vi "Get Autocomplete Search String.vi"(7 "String in":refnum<vi>, 11 "Autocomplete State in":T1) -> (2 "Search String":string, 3 "Autocomplete State out":T1)   [LabVIEW 2020, in "Output Sequencer.lvlib" / "Settings UI.lvclass"]
uses:
  Settings UI.lvclass
  Types/Autocomplete State.ctl
  Output Sequencer/Globals/Global Strings.vi
  Output Sequencer/Output Sequencer.lvclass
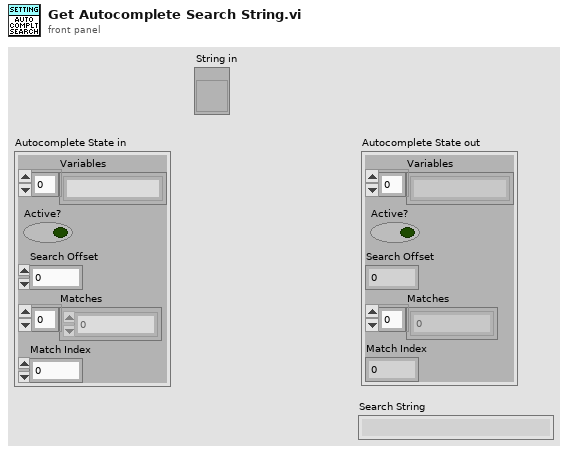
[diagram p1: front panel]
types:
  T1 = typedef "Output Sequencer.lvlib/Settings UI.lvclass/Autocomplete State.ctl" = cluster{"Variables":string[], "Active?":bool, "Search Offset":i32, "Matches":i32[], "Match Index":i32}
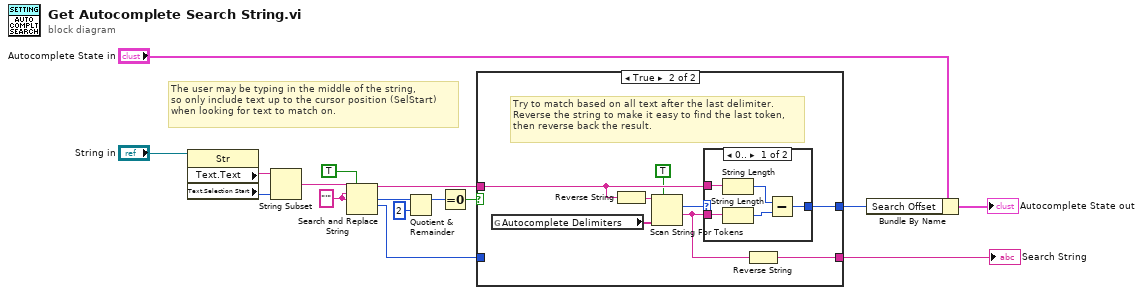
[diagram p0: block diagram]
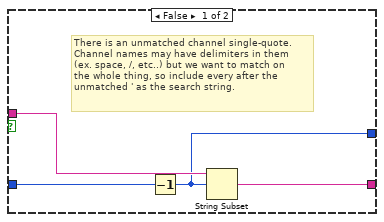
[diagram p2: hidden frame]
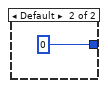
[diagram p3: hidden frame]
diagram:
  w12 = "'" ("search string")
  # "The user may be typing in the middle of the string,\nso only include text up to the cursor position (SelStart)\nwhen looking for text to match on."
  n1 = property class="Str"(reference="String in") -> ("Text.Text"=w5:string, "Text.Selection Start"=w4:u32)  [unwired: 1 in, 2 out]
  n2 = String Subset(string=w5, length (rest)=w4) -> (substring=w3:string)  [unwired: 1 in]
  n3 = Search and Replace String(replace all?=TRUE ("replace all? (F)"), input string=w3, search string=w12, replace string=w12) -> (result string=w10:string, number of replacements=w8:i32, offset past replacement=w7:i32)  [unwired: 4 in, 1 out]
  n4 = Quotient & Remainder(x=w8, y=2) -> (x-y*floor(x/y)=w2:i32)  [unwired: 1 out]
  n5 = Equal To 0?(x=w2) -> (x = 0?=w1:bool)
  n6 = case shown="True" w1 {
    tunnel: [w19 w28] -> w16
    tunnel: w10 -> [w20 w27]
    tunnel: w7 -> [w18 _]
    tunnel: [w17 w26] -> w6
    frame False {
      # "There is an unmatched channel single-quote.\nChannel names may have delimiters in them\n(ex. space, /, etc..) but we want to match on \nthe whole thing, so include every after the\nunmatched ' as the search string."
      n7 = Decrement(x=w18) -> (x-1=w17:i32)
      n8 = String Subset(string=w20, offset (0)=w17) -> (substring=w19:string)  [unwired: 1 in]
    }
    frame True {
      # "Try to match based on all text after the last delimiter.\nReverse the string to make it easy to find the last token,\nthen reverse back the result."
      n9 = global read "Global Strings.vi" "Autocomplete Delimiters"() -> (w25:string[])
      n10 = Reverse String(1:w27) -> (0:w21:string)
      n11 = Scan String For Tokens(5:TRUE ("allow empty tokens? (F)"), 6:w25, 9:w21) -> (1:w22:string, 2:w24:i32)  [unwired: 3 in, 2 out]
      n12 = case shown="0.." w24 {
        tunnel: w27 -> [w33 _]
        tunnel: [w31 0] -> w26
        tunnel: w22 -> [w30 _]
        frame 0.. {
          n13 = String Length(string=w33) -> (length=w32:i32)
          n14 = String Length(string=w30) -> (length=w29:i32)
          n15 = Subtract(x=w32, y=w29) -> (x-y=w31:i32)
        }
        frame Default {
        }
      }
      n16 = Reverse String(1:w22) -> (0:w28:string)
    }
  }
  "Search String" <- w16
  n17 = Bundle By Name(cluster="Autocomplete State in", "Search Offset"=w6) -> (→"Autocomplete State out":T1)
